vi "Control.vi"(8 "Control in":i32=2 format="%.3f", 9 "Sense":i32=2, 10 "Increment":dbl format="%.4f", 11 "Setpoint":i32=2) -> (2 "Overrange":bool, 3 "Control out":i32 format="%.3f")   [LabVIEW 2019]
doc: "This example demonstrates how to acquire a continuous amount of data (Waveform) using the DAQ device's internal clock. It also shows how to synchronize two devices for different device families (E Series, S Series, M Series, X Series, DSA, and SC Express), to simultaneously acquire the data.\n\nFor instructions on how to connect your signals to the DAQ device, refer to your device documentation."
panel:
  # "Control"
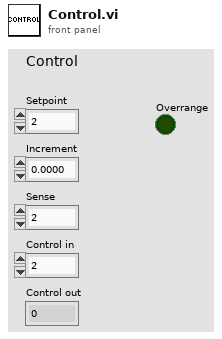
[diagram p1: front panel]
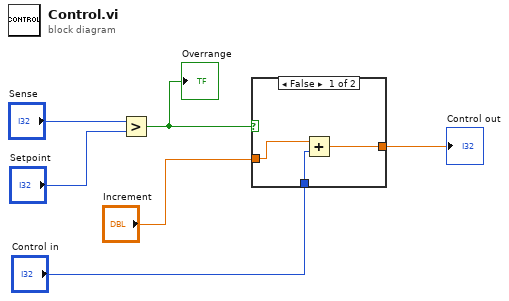
[diagram p0: block diagram]
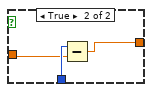
[diagram p2: hidden frame]
diagram:
  n1 = Greater?(x="Sense", y="Setpoint") -> (0:w4:bool)
  "Overrange" <- w4
  n2 = case shown="False" w4 {
    tunnel: "Control in" -> [w9 w12]
    tunnel: "Increment" -> [w8 w11]
    tunnel: [w7 w10] -> w1
    frame False {
      n3 = Add(x=w8, y=w9) -> (x+y=w7:dbl)
    }
    frame True {
      n4 = Subtract(x=w12, y=w11) -> (x-y=w10:dbl)
    }
  }
  "Control out" <- w1
